vi "Configure Trigger.vi"(5 "Slope (0: Negative)":u16(ring) items=["Negative", "Positive"], 6 "Manual Trigger Delay (0.0 s)":dbl format="%.5g", 7 "Internal Level (0)":dbl, 8 "error in (no error)":errorcluster, 9 "Enable Auto Delay (T: Enable)":bool=TRUE, 10 "Trigger Source (0: Immediate)":u16(ring) items=["Immediate", "Software (Bus)", "External", "Internal"], 11 "VISA resource name":refnum<visa-resource-name>) -> (0 "error out":errorcluster, 3 "VISA resource name out":refnum<visa-resource-name>)   [LabVIEW 2018, in "Agilent 34401.lvlib"]
doc: "Configures the trigger settings on the instrument.\n\n<B>Note:</B>\n\nThis VI will only be used with the low level Data VIs, as the high level VIs already contain this functionality."
uses:
  <instrlib>/Agilent 34401/Agilent 34401.lvlib
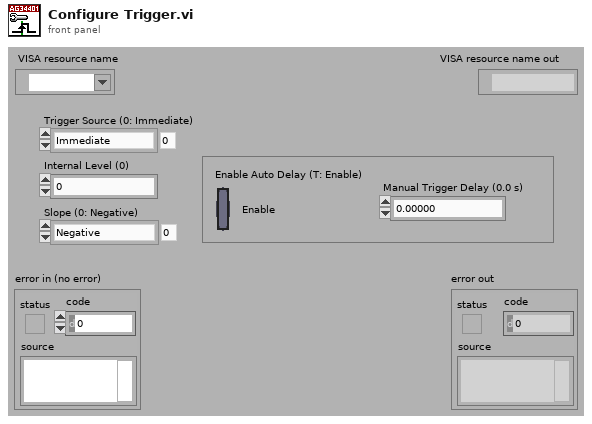
[diagram p1: front panel]
types:
  T1 = typedef "Agilent 34401.lvlib/Extended User Data.ctl" = cluster{"Trigger Source":u16, "Math Storage":u16, "Agilent Model":i32}
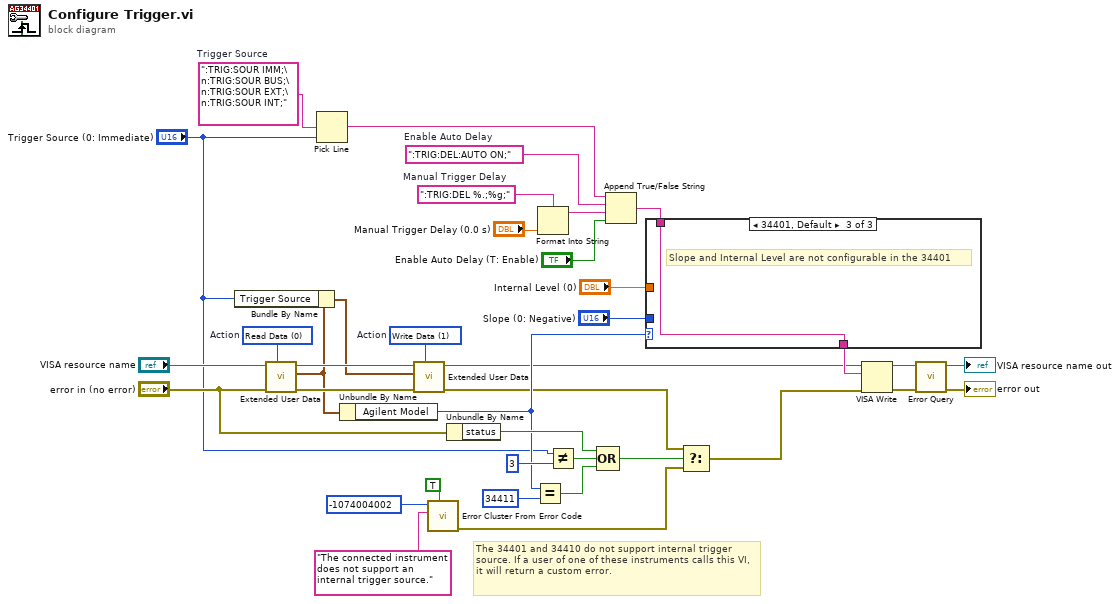
[diagram p0: block diagram]
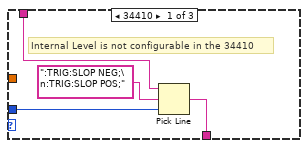
[diagram p2: hidden frame]
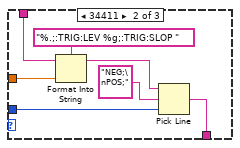
[diagram p3: hidden frame]
diagram:
  w11 = u16 0 items=["Read Data", "Write Data", "Dispose of Data"]  # Action
  w12 = u16 1 items=["Read Data", "Write Data", "Dispose of Data"]  # Action
  w30 = ":TRIG:DEL:AUTO ON;"  # Enable Auto Delay
  w31 = ":TRIG:DEL %.;%g;"  # Manual Trigger Delay
  w36 = ":TRIG:SOUR IMM;\n:TRIG:SOUR BUS;\n:TRIG:SOUR EXT;\n:TRIG:SOUR INT;"  # Trigger Source
  # "The 34401 and 34410 do not support internal trigger source. If a user of one of these instruments calls this VI, it will return a custom error."
  n1 = call <instrlib>:"Extended User Data.vi"("Action (0: Read Data)"=w11, "Error In (no error)"="error in (no error)", "VISA resource name in"="VISA resource name") -> ("Error Out"=w10:errorcluster, "User Data Out"=w1:T1, "VISA resource name out"=w9:refnum<visa-resource-name>)  [unwired: 6 in]
  n2 = Bundle By Name(cluster=w1, "Trigger Source"="Trigger Source (0: Immediate)") -> (w3:T1)
  n3 = Pick Line(multi-line string=w36, line index="Trigger Source (0: Immediate)") -> (output string=w28:string)  [unwired: 1 in]
  n4 = Unbundle By Name(w1) -> ("Agilent Model"=w6:i32)
  n5 = call <instrlib>:"Extended User Data.vi"("Action (0: Read Data)"=w12, "Error In (no error)"=w10, "User Data In"=w3, "VISA resource name in"=w9) -> ("Error Out"=w4:errorcluster, "VISA resource name out"=w5:refnum<visa-resource-name>)  [unwired: 5 in, 1 out]
  n6 = call <vilib>:"Error Cluster From Error Code.vi"("show call chain? (False)"=TRUE, "error message (\"\")"="The connected instrument does not support an internal trigger source." ("Source (VI Name)"), "error code (0)"=-1074004002 ("Code")) -> ("error out"=w18:errorcluster)  [unwired: 6 in]
  n7 = Unbundle By Name("error in (no error)") -> ("status"=w15:bool)
  n8 = Equal?(x=w6, y=u32 34411) -> (x = y?=w14:bool)
  n9 = Format Into String(format string=w31, "Manual Trigger Delay (0.0 s)") -> (resulting string=w29:string)  [unwired: 2 in, 1 out]
  n10 = Not Equal?(x="Trigger Source (0: Immediate)", y=u16 3) -> (x != y?=w16:bool)
  n11 = Compound Arithmetic op=OR(w15, w16, w14) -> (w19:bool)
  n12 = Append True/False String(1:"Enable Auto Delay (T: Enable)", 2:w29, 3:w30, 4:w28) -> (0:w27:string)
  n13 = case shown="34401, Default" w6 {
    tunnel: w27 -> [w40 w49 w50]
    tunnel: [w39 w45 w50] -> w26
    tunnel: "Internal Level (0)" -> [_ w48 _]
    tunnel: "Slope (0: Negative)" -> [w42 w43 _]
    frame 34410 {
      # "Internal Level is not configurable in the 34410"
      n14 = Pick Line(string ("")=w40, multi-line string=":TRIG:SLOP NEG;\n:TRIG:SLOP POS;" ("true string"), line index=w42) -> (output string=w39:string)
    }
    frame 34411 {
      n15 = Format Into String(format string="%.;:TRIG:LEV %g;:TRIG:SLOP ", initial string=w49, w48) -> (resulting string=w46:string)  [unwired: 1 in, 1 out]
      n16 = Pick Line(string ("")=w46, multi-line string="NEG;\nPOS;" ("true string"), line index=w43) -> (output string=w45:string)
    }
    frame 34401, Default {
      # "Slope and Internal Level are not configurable in the 34401"
    }
  }
  n17 = Select(t=w4, s=w19, f=w18) -> (s? t:f=w17:errorcluster)
  n18 = VISA Write(VISA resource name=w5, write buffer=w26, error in (no error)=w17) -> (VISA resource name out=w35:refnum<visa-resource-name>, error out=w34:errorcluster)  [unwired: 1 out]
  n19 = call <instrlib>:"Error Query.vi"("error in (no error)"=w34, "VISA resource name"=w35) -> ("error out"=→"error out":errorcluster, "VISA resource name out"=→"VISA resource name out":refnum<visa-resource-name>)  [unwired: 6 in, 2 out]
